vi "DrawBackground.vi"(8 "error in (no error)":errorcluster, 11 "Menu in":refnum<class "Menu.lvclass">) -> (0 "error out":errorcluster, 3 "Menu out":refnum<class "Menu.lvclass">)   [LabVIEW 2019, in "RT_Game.lvlib" / "Menu.lvclass"]
uses:
  Menu.lvclass
  C:/Users/FreshBob/Dropbox/VIs/myRIO_GameConsole/RT/RT_Game/Game/Game.lvclass
  Menu.lvclass/Menu.ctl
  Game/Game.lvclass
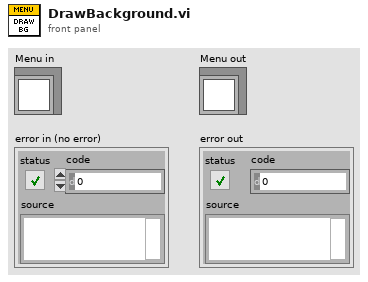
[diagram p1: front panel]
types:
  T1 = typedef "RT_Game.lvlib/Game.lvclass/Coordinate.ctl" = cluster{"x":dbl, "y":dbl}
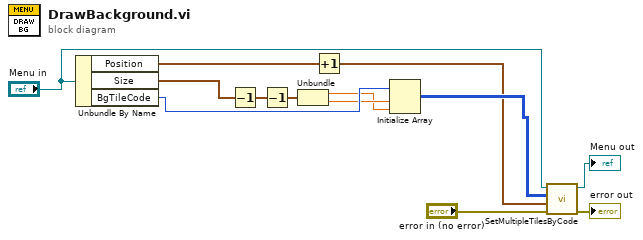
[diagram p0: block diagram]
diagram:
  n1 = Unbundle By Name("Menu in") -> ("Position"=w12:T1, "Size"=w2:T1, "BgTileCode"=w8:u32)
  n2 = Decrement(x=w2) -> (x-1=w1:T1)
  n3 = Decrement(x=w1) -> (x-1=w3:T1)
  n4 = Unbundle(w3) -> ("x"=w6:dbl, "y"=w7:dbl)
  n5 = Increment(x=w12) -> (x+1=w4:T1)
  n6 = Initialize Array(w8, w7, w6) -> (w5:u32[][])
  n7 = call "SetMultipleTilesByCode.vi"("error in (no error)"="error in (no error)", "Position"=w4, "TileCodes"=w5, "Game in"="Menu in") -> ("error out"=→"error out":errorcluster, "Game out"=→"Menu out":refnum<class "Menu.lvclass">)  [unwired: 6 in]
